vi "Get Full Decay Fit & Residual Plots (2-Exp Fit) v2.vi"(4 "SYNC Period":dbl[unit], 6 "Fit Options":T2={"Show Fit Residuals"=TRUE, "Fit Model"=enum."1-Exponential", "Residual Type"=enum."Standard", "Max Decay Percentile"=0.0, "Min Decay Percentile"=0.0, "Show Full Decay"=TRUE, "Weights"=enum."Unweighted", "Fitting Method"=enum."Least Square", "Compute Parameter Uncertainties"=TRUE, "Periodic Boundaries"=TRUE, "Model Calculation"=enum."Simulation", "Period"=1.2500000000000001e-08, "Termination Criteria"={"Max Iterations"=1000, "Max Function Calls"=0, "Max Time"=1000.0, "Function Tolerance"=1e-06, "Parameter Tolerance"=1e-06, "Gradient Tolerance"=0.0, "Min Lambda"=1e-06, "Max Lambda"=1e-06, "Initial Tick Count"=0}, "Offset Resolution"=1.2500000000000001e-08, "Use Local IRF"=TRUE, "Fitting Algorithm"=enum."Levenberg-Marquardt", "Show Confidence Interval "=TRUE, "Confidence Level"=95.0} {"Confidence Level" min=0.0 max=100.0; "Offset Resolution" min=0.0; "Period" min=0.0; "Min Decay Percentile" min=0.0 max=1.0; "Max Decay Percentile" min=0.0 max=100.0}, 7 "Use Normalized IRF (T)":bool=TRUE, 8 "Error In":errorcluster, 9 "Best Fit Parameters (w tau)":dbl[](array[numeric]), 10 "IRF":cluster{"t Array":dbl[], "IRF Array":dbl[]}, 11 "Full Decay":cluster{"t Array":dbl[], "Y Array":dbl[]}) -> (0 "Error Out":errorcluster, 3 "Fit Plots":T1)   [LabVIEW 2021, in "Fits.lvlib"]
uses:
  Fits.lvlib
  Decay Convolution/Decay Model.ctl
  Residual Type.ctl
  Non-linear Fitting Method v2.ctl
  Fit Calculation Method.ctl
  Non-linear Fitting Algorithm.ctl
  Fit Plots.ctl
  <vilib>/gmath/NumericalOptimization/LM_output select.ctl
  Decay Convolution/Fit Control Data v2.ctl
  Graphs/XY Graph/XY Graph Plot Data.ctl
  Decay Fit Parameters In List.ctl
  Decay Convolution/Fit Control Data.ctl
  Graphs/XY Graph/XY Graph Add-Ons.lvlib
  <vilib>/gmath/NI_Gmath.lvlib
  Fit Weights Type v2.ctl
  Decay Fit Options v4.ctl
panel:
  out "XY Graph":cluster{"t Array":dbl[], "f(X,a)":dbl[]}[](graph)
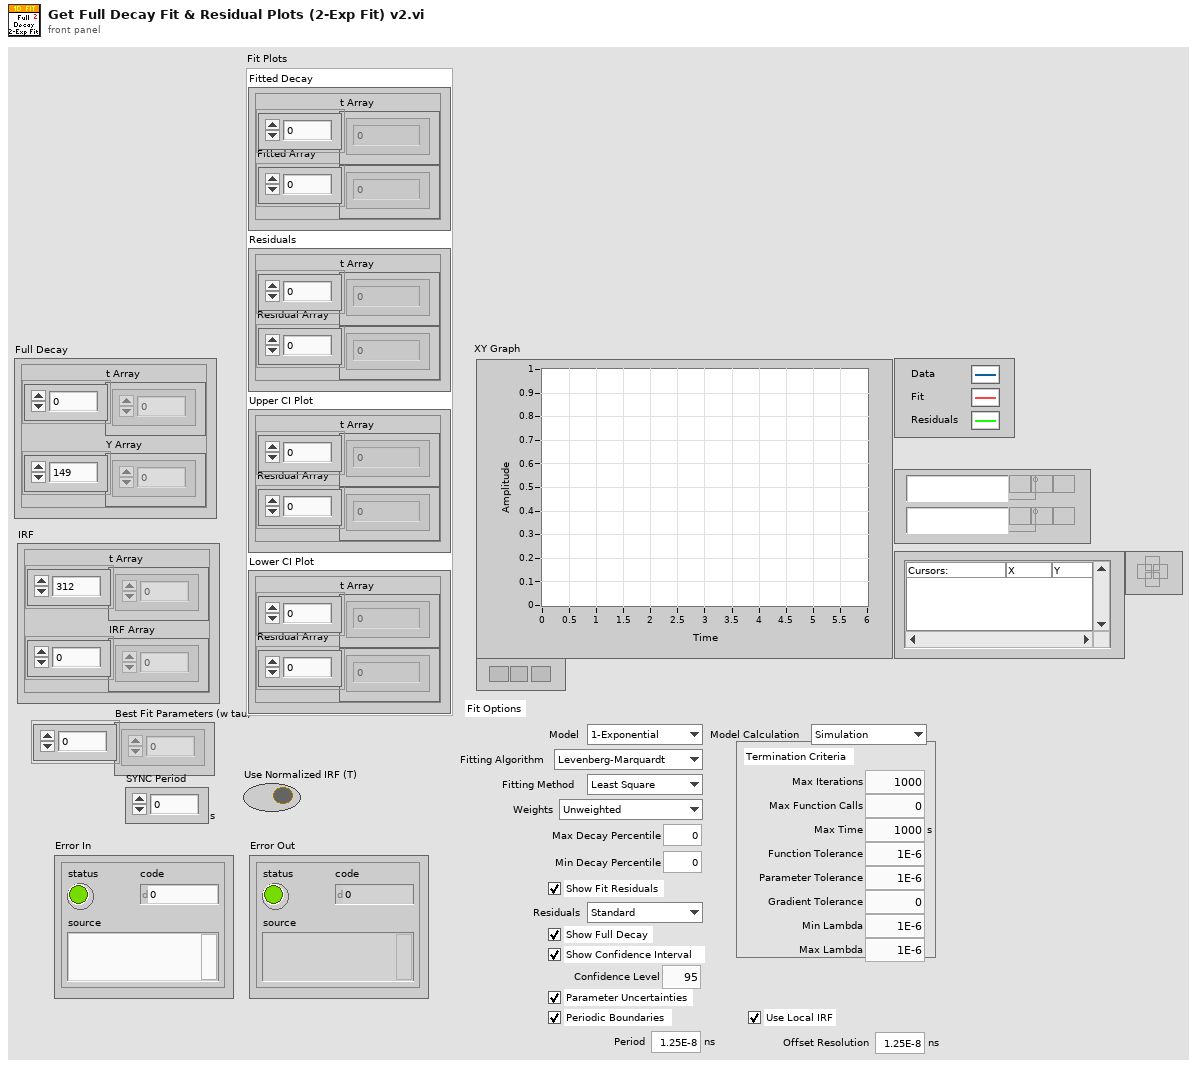
[diagram p1: front panel]
types:
  T1 = typedef "Fits.lvlib/Fit Plots.ctl" = cluster{"Fitted Decay":cluster{"t Array":dbl[], "Fitted Array":dbl[]}, "Residuals":cluster{"t Array":dbl[], "Residual Array":dbl[]}, "Upper CI Plot":cluster{"t Array":dbl[], "Residual Array":dbl[]}, "Lower CI Plot":cluster{"t Array":dbl[], "Residual Array":dbl[]}}
  T2 = typedef "Fits.lvlib/Decay Fit Options v4.ctl" = cluster{"Show Fit Residuals":bool, "Fit Model":T3, "Residual Type":T4, "Max Decay Percentile":dbl, "Min Decay Percentile":dbl, "Show Full Decay":bool, "Weights":T5, "Fitting Method":T6, "Compute Parameter Uncertainties":bool, "Periodic Boundaries":bool, "Model Calculation":T7, "Period":dbl[unit], "Termination Criteria":cluster{"Max Iterations":i32, "Max Function Calls":i32, "Max Time":dbl[unit], "Function Tolerance":dbl, "Parameter Tolerance":dbl, "Gradient Tolerance":dbl, "Min Lambda":dbl, "Max Lambda":dbl, "Initial Tick Count":u32}, "Offset Resolution":dbl[unit], "Use Local IRF":bool, "Fitting Algorithm":T8, "Show Confidence Interval ":bool, "Confidence Level":dbl}
  T3 = typedef "Fits.lvlib/Decay Model.ctl" = enum16{"1-Exponential", "2-Exponentials"}
  T4 = typedef "Fits.lvlib/Residual Type.ctl" = enum16{"Standard", "Normalized", "Reduced"}
  T5 = typedef "Fits.lvlib/Fit Weights Type v2.ctl" = enum16{"Unweighted", "1/Variance (Neyman)", "1/Variance (Pearson)", "Best of All"}
  T6 = typedef "Fits.lvlib/Non-linear Fitting Method v2.ctl" = enum16{"Least Square", "Least Absolute Residual", "Bisquare", "MLE", "-", "Best of All"}
  T7 = typedef "Fits.lvlib/Fit Calculation Method.ctl" = enum16{"Simulation", "Convolution", "Integration"}
  T8 = typedef "Fits.lvlib/Non-linear Fitting Algorithm.ctl" = enum16{"Levenberg-Marquardt", "Trust-Region Dogleg"}
  T9 = typedef "Fits.lvlib/Fit Control Data.ctl" = cluster{"IRF":T10, "Laser Period":dbl, "SYNC Period":dbl}
  T10 = typedef "XY Graph Add-Ons.lvlib/XY Graph Plot Data.ctl" = cluster{"X Array":dbl[], "Y Array":dbl[]}
  T11 = typedef "Fits.lvlib/Fit Control Data v2.ctl" = cluster{"IRF":T10, "Laser Period":dbl, "SYNC Period":dbl, "Fixed Parameter Names":T12[], "Fixed Parameter Values":dbl[], "Fitted Parameter Names":T12[], "Fit Model":T3}
  T12 = typedef "Fits.lvlib/Decay Fit Parameters In List.ctl" = enum16{"Offset", "Baseline", "A_1", "tau_1", "A_2", "tau_2"}
  T13 = typedef "NI_Gmath.lvlib/LM_output select.ctl" = cluster{"model function":bool, "gradient":bool}
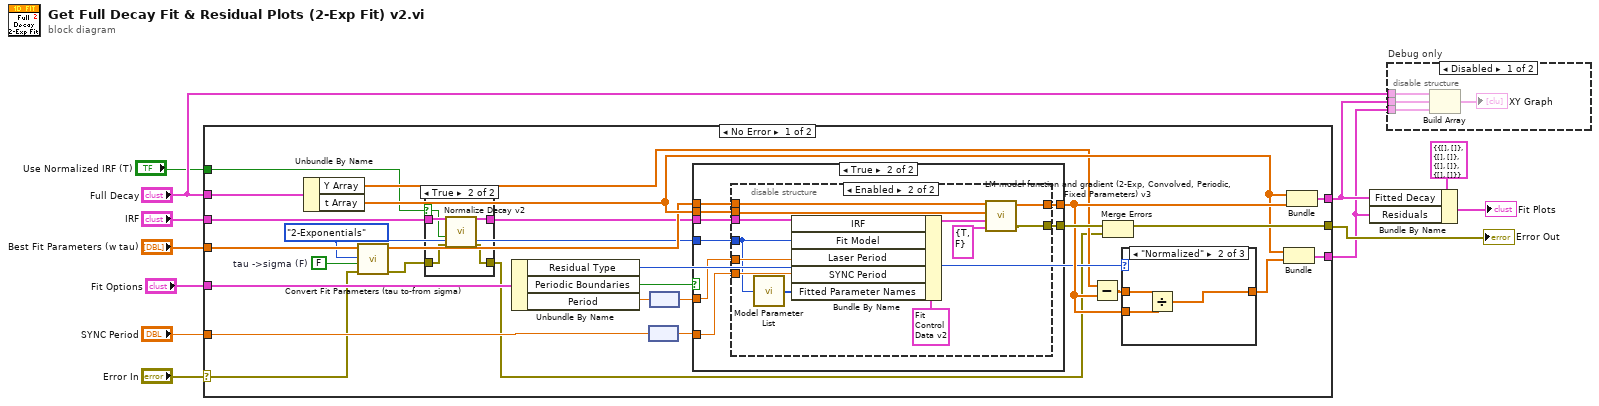
[diagram p0: block diagram]
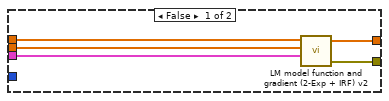
[diagram p4: hidden frame]
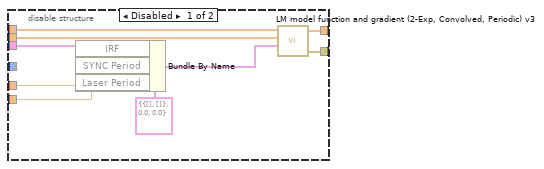
[diagram p5: hidden frame]
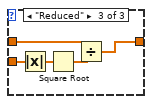
[diagram p7: hidden frame]
diagram:
  n1 = case shown="No Error" "Error In" {
    selector: "Error In" -> [w19 w90]
    tunnel: "IRF" -> [w17 _]
    tunnel: "Best Fit Parameters (w tau)" -> [w22 _]
    tunnel: [w39 _] -> w2
    tunnel: [w32 w90] -> w9
    tunnel: [w36 _] -> w1
    tunnel: "Full Decay" -> [w34 _]
    tunnel: "SYNC Period" -> [w31 _]
    tunnel: "Fit Options" -> [w30 _]
    tunnel: "Use Normalized IRF (T)" -> [w15 _]
    frame No Error {
      w18 = Decay_Model."2-Exponentials" ("Fit Model")
      w21 = FALSE  # tau ->sigma (F)
      n2 = Unbundle By Name(w34) -> ("Y Array"=w23:dbl[], "t Array"=w25:dbl[])
      n3 = call "Convert Fit Parameters (tau to-from sigma).vi"("Error In"=w19, "tau ->sigma (F)/sigma->tau (T)"=w21, "Fit Model"=w18, "All Parameters in"=w22) -> ("Error Out"=w14:errorcluster, "All Parameters out"=w20:dbl[])  [unwired: 6 in]
      n4 = case shown="True" w15 {
        selector: w15 -> [_ w42]
        tunnel: w17 -> [w41 w46]
        tunnel: [w41 w45] -> w16
        tunnel: w14 -> [w40 w44]
        tunnel: [w40 w43] -> w13
        frame False {
        }
        frame True {
          n5 = call "Normalize Decay v2.vi"("Error In"=w44, "Max = 1 (F)/Integral = 1 (T)"=w42, "Decay"=w46) -> ("Error Out"=w43:errorcluster, "Normalized Decay"=w45:cluster{"t Array":dbl[], "Y Array":dbl[]})  [unwired: 4 in, 3 out]
        }
      }
      n6 = Unbundle By Name(w30) -> ("Residual Type"=w24:T4, "Periodic Boundaries"=w29:bool, "Period"=w27:dbl[unit])
      n7 = node(w31) -> (w28:dbl)
      n8 = node(w27) -> (w26:dbl)
      n9 = case shown="True" w29 {
        tunnel: [w51 w56] -> w38
        tunnel: [w50 w57] -> w35
        tunnel: w16 -> [w49 w55]
        tunnel: w20 -> [w48 w59]
        tunnel: w25 -> [w47 w58]
        tunnel: w28 -> [_ w54]
        tunnel: w26 -> [_ w53]
        tunnel: w18 -> [_ w52]
        frame False {
          n10 = call "LM model function and gradient (2-Exp + IRF) v2.vi"("data"=w49, "X"=w47, "a"=w48) -> ("error out"=w51:errorcluster, "f(X,a)"=w50:dbl[])  [unwired: 1 in, 1 out]
        }
        frame True {
          n11 = disable-structure shown="Enabled" {
            disable-tunnel: w59 -> [w68 w80]
            disable-tunnel: w58 -> [w67 w79]
            disable-tunnel: [w66 w76] -> w57
            disable-tunnel: [w65 w77] -> w56
            disable-tunnel: w55 -> [w64 w75]
            disable-tunnel: w54 -> [w61 w73]
            disable-tunnel: w53 -> [w60 w74]
            disable-tunnel: w52 -> [_ w71]
            frame Disabled {
              n12 = Bundle By Name(cluster=T9 {"IRF"={"X Array"=[], "Y Array"=[]}, "Laser Period"=0.0, "SYNC Period"=0.0} ("Fit Control Data"), "IRF"=w64, "SYNC Period"=w60, "Laser Period"=w61) -> (w62:T9)
              n13 = call "LM model function and gradient (2-Exp, Convolved, Periodic) v3.vi"("data"=w62, "X"=w67, "a"=w68) -> ("error out"=w65:errorcluster, "f(X,a)"=w66:dbl[])  [unwired: 1 in, 1 out]
            }
            frame Enabled {
              n14 = call "Model Parameter List.vi"("Fit Model"=w71) -> ("Model Parameter List"=w70:T12[])
              n15 = Bundle By Name(cluster=T11 {"IRF"={"X Array"=[], "Y Array"=[]}, "Laser Period"=0.0, "SYNC Period"=0.0, "Fixed Parameter Names"=[], "Fixed Parameter Values"=[], "Fitted Parameter Names"=[], "Fit Model"=enum."1-Exponential"} ("Fit Control Data"), "IRF"=w75, "Fit Model"=w71, "Laser Period"=w74, "SYNC Period"=w73, "Fitted Parameter Names"=w70) -> (w69:T11)
              n16 = call "LM model function and gradient (2-Exp, Convolved, Periodic, Fixed Parameters) v3.vi"("output control"=T13 {"model function"=TRUE, "gradient"=FALSE}, "data"=w69, "X"=w79, "a (with sigma)"=w80) -> ("error out"=w77:errorcluster, "f(X,a)"=w76:dbl[])  [unwired: 1 out]
            }
          }
        }
      }
      n17 = Subtract(x=w23, y=w35) -> (x-y=w33:dbl[])
      n18 = Merge Errors(w38, w13) -> (w32:errorcluster)
      n19 = case shown="\"Normalized\"" w24 {
        tunnel: w33 -> [w81 w84 w89]
        tunnel: [w81 w82 w87] -> w37
        tunnel: w35 -> [_ w83 w88]
        frame "Standard", Default {
        }
        frame "Normalized" {
          n20 = Divide(x=w84, y=w83) -> (x/y=w82:dbl[])
        }
        frame "Reduced" {
          n21 = Absolute Value(x=w88) -> (abs(x)=w86:dbl[])
          n22 = Square Root(x=w86) -> (sqrt(x)=w85:dbl[])
          n23 = Divide(x=w89, y=w85) -> (x/y=w87:dbl[])
        }
      }
      n24 = Bundle("t Array"=w25, w37) -> (w36:cluster{"t Array":dbl[], dbl[]})  [unwired: 1 in]
      n25 = Bundle("t Array"=w25, "f(X,a)"=w35) -> (w39:cluster{"t Array":dbl[], "f(X,a)":dbl[]})  [unwired: 1 in]
    }
    frame Error {
    }
  }
  "Error Out" <- w9
  n26 = Bundle By Name(cluster=T1 {"Fitted Decay"={"t Array"=[], "Fitted Array"=[]}, "Residuals"={"t Array"=[], "Residual Array"=[]}, "Upper CI Plot"={"t Array"=[], "Residual Array"=[]}, "Lower CI Plot"={"t Array"=[], "Residual Array"=[]}} ("Fit Plots"), "Fitted Decay"=w2, "Residuals"=w1) -> (→"Fit Plots":T1)
  n27 = disable-structure "Debug only" shown="Disabled" {
    disable-tunnel: "Full Decay" -> [w94 _]
    disable-tunnel: w2 -> [w92 _]
    disable-tunnel: w1 -> [w91 _]
    frame Disabled {
      n28 = Build Array(w94, w92, w91) -> (→"XY Graph":cluster{"t Array":dbl[], "f(X,a)":dbl[]}[])
    }
    frame Enabled {
    }
  }
